vi "fileDelete.vi"   [LabVIEW 2017]
doc: "Checks if any frame has been saved. If not, it deletes the whole folder to remove the clutter."
uses:
  globalUtilities.vi
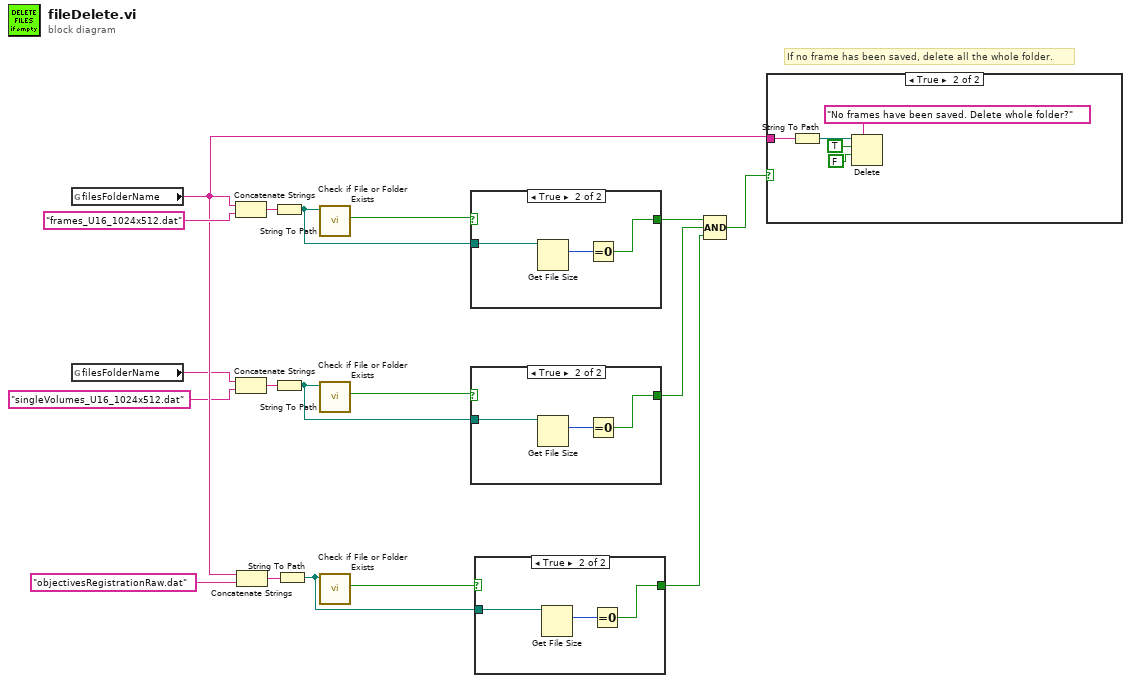
[diagram p0: block diagram]
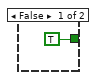
[diagram p2: hidden frame]
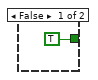
[diagram p3: hidden frame]
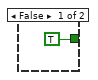
[diagram p4: hidden frame]
diagram:
  # "If no frame has been saved, delete all the whole folder."
  n1 = global read "globalUtilities.vi" "filesFolderName"() -> (w14:string)
  n2 = global read "globalUtilities.vi" "filesFolderName"() -> (w7:string)
  n3 = Concatenate Strings(w14, "frames_U16_1024x512.dat") -> (w17:string)
  n4 = Concatenate Strings(w7, "singleVolumes_U16_1024x512.dat") -> (w4:string)
  n5 = Concatenate Strings(w14, "objectivesRegistrationRaw.dat" ("string")) -> (w12:string)
  n6 = String To Path(string=w17) -> (path=w15:path)
  n7 = String To Path(string=w4) -> (path=w6:path)
  n8 = String To Path(string=w12) -> (path=w10:path)
  n9 = call <vilib>:"Check if File or Folder Exists.vi"("path"=w15) -> ("file or folder exists?"=w16:bool)  [unwired: 8 in, 2 out]
  n10 = call <vilib>:"Check if File or Folder Exists.vi"("path"=w6) -> ("file or folder exists?"=w5:bool)  [unwired: 8 in, 2 out]
  n11 = call <vilib>:"Check if File or Folder Exists.vi"("path"=w10) -> ("file or folder exists?"=w11:bool)  [unwired: 8 in, 2 out]
  n12 = case shown="True" w16 {
    tunnel: [TRUE w21] -> w9
    tunnel: w15 -> [_ w20]
    frame False {
    }
    frame True {
      n13 = Get File Size(file=w20) -> (size (in bytes)=w22:i64)  [unwired: 1 in, 2 out]
      n14 = Equal To 0?(x=w22) -> (x = 0?=w21:bool)
    }
  }
  n15 = case shown="True" w5 {
    tunnel: [TRUE w25] -> w1
    tunnel: w6 -> [_ w24]
    frame False {
    }
    frame True {
      n16 = Get File Size(file=w24) -> (size (in bytes)=w26:i64)  [unwired: 1 in, 2 out]
      n17 = Equal To 0?(x=w26) -> (x = 0?=w25:bool)
    }
  }
  n18 = case shown="True" w11 {
    tunnel: [TRUE w29] -> w2
    tunnel: w10 -> [_ w28]
    frame False {
    }
    frame True {
      n19 = Get File Size(file=w28) -> (size (in bytes)=w30:i64)  [unwired: 1 in, 2 out]
      n20 = Equal To 0?(x=w30) -> (x = 0?=w29:bool)
    }
  }
  n21 = Compound Arithmetic op=AND(w9, w1, w2) -> (w8:bool)
  n22 = case shown="True" w8 {
    tunnel: w14 -> [_ w35]
    frame False {
    }
    frame True {
      n23 = String To Path(string=w35) -> (path=w34:path)
      n24 = Delete(prompt (Delete)="No frames have been saved. Delete whole folder?", path (use dialog)=w34, entire hierarchy (F)=TRUE, confirm (F)=FALSE) -> ()  [unwired: 1 in, 3 out]
    }
  }
